vi "Symphony Setup.vi"(0 "JYCCDLib.IJYCCDReqd":refnum<k7>, 1 "ADC":i32(ring) items=["JY_ADC_16_BIT", "JY_ADC_14_BIT", "JY_ADC_18_BIT"], 5 "Image Mode":bool caption="Image Mode?", 7 "Integration (s)":dbl=10.0, 9 "Symphony Area Format":T1, 11 "Error Input":errorcluster, 12 "Gain":i32) -> (4 "DataSize":i32, 15 "Error Output":errorcluster caption="Error Ouput")   [LabVIEW 2010]
uses:
  TypeDefs/Symphony Area Format.ctl
panel:
  out "XSize":i32
  out "YSize":i32
  out "XBin":i32
  out "YBin":i32
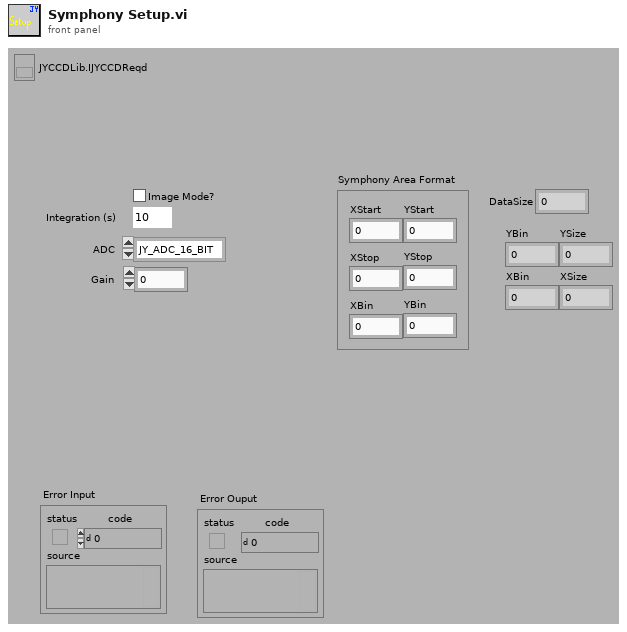
[diagram p1: front panel]
types:
  T1 = typedef "Symphony Area Format.ctl" = cluster{"XStart":i32, "YStart":i32, "XStop":i32, "YStop":i32, "XBin":i32, "YBin":i32}
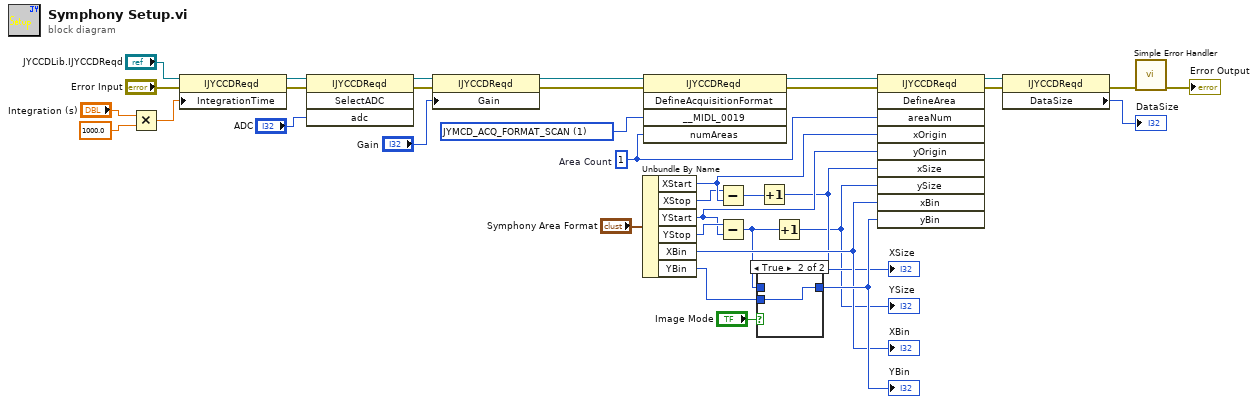
[diagram p0: block diagram]
diagram:
  w29 = 1 items=["JYMCD_ACQ_FORMAT_IMAGE", "JYMCD_ACQ_FORMAT_SCAN"] ("Acq. Type")
  w16 = 1  # Area Count
  n1 = Multiply(x="Integration (s)", y=1000.0) -> (x*y=w9:dbl)
  n2 = property class="IJYCCDReqd"(reference="JYCCDLib.IJYCCDReqd", error in="Error Input", "IntegrationTime"=w9) -> (reference out=w31:refnum<k7>, error out=w35:errorcluster)
  n3 = invoke class="IJYCCDReqd" method="SelectADC"(reference=w31, error in=w35, "adc"="ADC") -> (reference out=w30:refnum<k7>, error out=w34:errorcluster)  [unwired: 1 in, 2 out]
  n4 = property class="IJYCCDReqd"(reference=w30, error in=w34, "Gain"="Gain") -> (reference out=w28:refnum<k7>, error out=w27:errorcluster)
  n5 = Unbundle By Name("Symphony Area Format") -> ("XStart"=w8:i32, "XStop"=w7:i32, "YStart"=w5:i32, "YStop"=w6:i32, "XBin"=w12:i32, "YBin"=w13:i32)
  "XBin" <- w12
  n6 = invoke class="IJYCCDReqd" method="DefineAcquisitionFormat"(reference=w28, error in=w27, "__MIDL_0019"=w29, "numAreas"=w16) -> (reference out=w26:refnum<k7>, error out=w22:errorcluster)  [unwired: 1 in, 3 out]
  n7 = Subtract(x=w7, y=w8) -> (x-y=w4:i32)
  n8 = Subtract(x=w6, y=w5) -> (x-y=w1:i32)
  n9 = case shown="True" "Image Mode" {
    tunnel: w1 -> [w36 _]
    tunnel: [w36 w37] -> w14
    tunnel: w13 -> [_ w37]
    frame False {
    }
    frame True {
    }
  }
  "YBin" <- w14
  n10 = Increment(x=w4) -> (x+1=w3:i32)
  "XSize" <- w3
  n11 = Increment(x=w1) -> (x+1=w2:i32)
  "YSize" <- w2
  n12 = invoke class="IJYCCDReqd" method="DefineArea"(reference=w26, error in=w22, "areaNum"=w16, "xOrigin"=w8, "yOrigin"=w5, "xSize"=w3, "ySize"=w2, "xBin"=w12, "yBin"=w14) -> (reference out=w25:refnum<k7>, error out=w24:errorcluster)  [unwired: 1 in, 8 out]
  n13 = property class="IJYCCDReqd"(reference=w25, error in=w24) -> (error out=w20:errorcluster, "DataSize"=→"DataSize":i32)  [unwired: 1 out]
  n14 = call <vilib>:"Simple Error Handler.vi"("error in (no error)"=w20) -> ("error out"=→"Error Output":errorcluster)  [unwired: 1 in, 7 out]
